vi "Call Geneaology Script.vi"(0 "PN":string, 7 "SN":string, 11 "Error In":errorcluster) -> (2 "Success":bool, 4 "Console Text":string, 15 "Error Out":errorcluster)   [LabVIEW 2021]
doc: "Calls the Python script to run the uds geneaology."
uses:
  <vilib>/regexp/Match Regular Expression.xnode
panel:
  # "Inputs"
  # "Outputs"
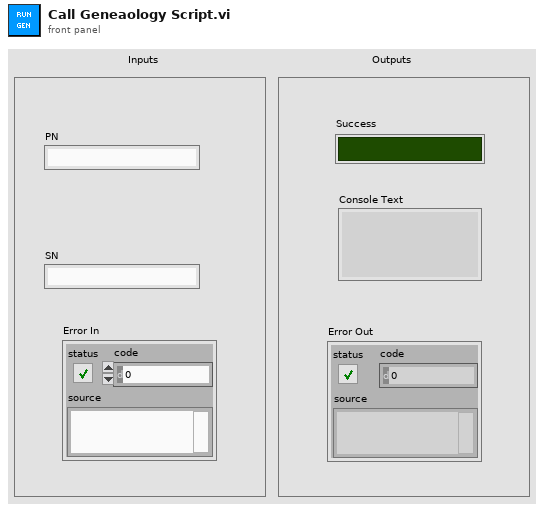
[diagram p1: front panel]
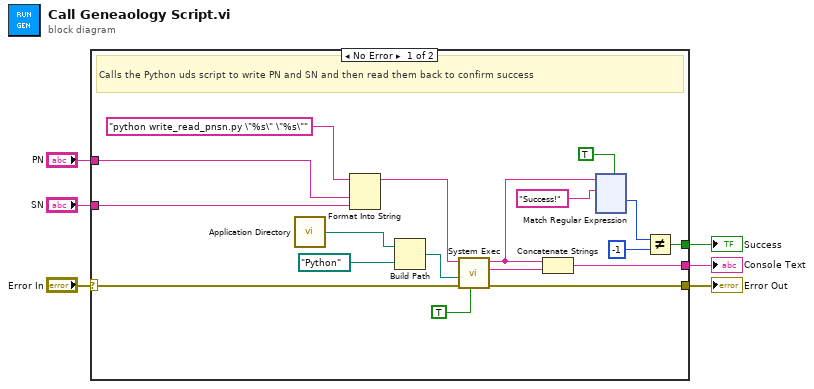
[diagram p0: block diagram]
diagram:
  n1 = case shown="No Error" "Error In" {
    selector: "Error In" -> [w24 w142]
    tunnel: [w17 w142] -> w5
    tunnel: [w15 _] -> w4
    tunnel: [w13 _] -> w3
    tunnel: "PN" -> [w8 _]
    tunnel: "SN" -> [w7 _]
    frame No Error {
      # "Calls the Python uds script to write PN and SN and then read them back to confirm success"
      n2 = call <vilib>:"Application Directory.vi"() -> ("Application Directory"=w23:path)
      n3 = Format Into String(format string="python write_read_pnsn.py \"%s\" \"%s\"" ("command line"), w8, w7) -> (resulting string=w9:string)  [unwired: 2 in, 1 out]
      n4 = Build Path(base path=w23, name or relative path=path "Python") -> (appended path=w21:path)
      n5 = call <vilib>:"System Exec.vi"("run minimized? (F)"=TRUE, "error in (no error)"=w24, "working directory"=w21, "command line"=w9) -> ("error out"=w17:errorcluster, "standard error"=w14:string, "standard output"=w16:string)  [unwired: 4 in, 1 out]
      n6 = Concatenate Strings(w16, w14) -> (w15:string)
      n7 = xnode "Match Regular Expression"("input string"=w16, "regular expression"="Success!" ("search string/char (-)"), "multiline? (F)"=TRUE) -> ("offset past match"=w11:i32)  [unwired: 3 in, 4 out]
      n8 = Not Equal?(x=w11, y=-1 ("x")) -> (x != y?=w13:bool)
    }
    frame Error {
      # "Can't start due to error"
    }
  }
  "Error Out" <- w5
  "Success" <- w3
  "Console Text" <- w4
